vi "Co-Pilot Teleop Cmd Changed.vi"(0 "New_Co-Pilot Data":T1, 2 "Co-Pilot Data":T1, 3 "Epsilon":dbl) -> (6 "Boolean":bool)   [LabVIEW 2014]
uses:
  Co-Pilot_game_control.ctl
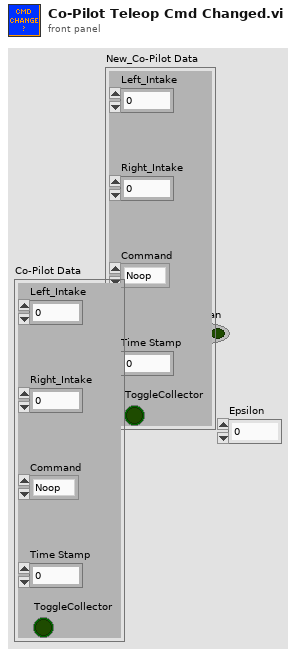
[diagram p1: front panel]
types:
  T1 = typedef "Co-Pilot_game_control.ctl" = cluster{"Left_Intake":dbl, "Right_Intake":dbl, "Time Stamp":u32, "Command":enum16{"Noop", "Flagged"}, "ToggleCollector":bool}
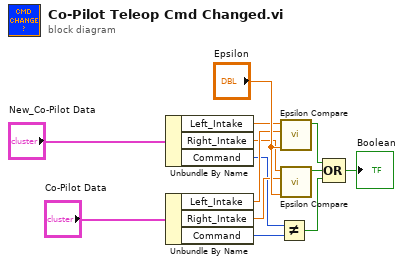
[diagram p0: block diagram]
diagram:
  n1 = Unbundle By Name("New_Co-Pilot Data") -> ("Left_Intake"=w7:dbl, "Right_Intake"=w5:dbl, "Command"=w3:enum16{"Noop", "Flagged"})
  n2 = Unbundle By Name("Co-Pilot Data") -> ("Left_Intake"=w6:dbl, "Right_Intake"=w4:dbl, "Command"=w2:enum16{"Noop", "Flagged"})
  n3 = Not Equal?(x=w3, y=w2) -> (x != y?=w1:bool)
  n4 = call "Epsilon Compare.vi"("Epsilon"="Epsilon", "Value2"=w6, "Value1"=w7) -> ("Boolean"=w12:bool)  [unwired: 8 in]
  n5 = call "Epsilon Compare.vi"("Epsilon"="Epsilon", "Value2"=w4, "Value1"=w5) -> ("Boolean"=w11:bool)  [unwired: 8 in]
  n6 = Compound Arithmetic op=OR(w12, w11, w1) -> (→"Boolean":bool)
